vi "Make Config File Body.vi"(0 "VISA resource name":refnum<visa-resource-name>, 11 "error in (no error)":errorcluster) -> (4 "VISA resource name out":refnum<visa-resource-name>, 6 "Result":string, 15 "error out":errorcluster)   [LabVIEW 2020, in "Yokogawa GX Series.lvlib"]
doc: "This VI sets the alarm hysteresis for <B>DX1000/DX2000 series</B>.\nThis VI can be used on Basic Setting Mode at the <B>Set Execution Mode.VI</B>.\n\nAlarm settings on computation channels can be specified on models with the /M1 or /PM1 math option.\nAlarm settings on external input channels can be specified on models with the /MC1 external input channel option."
uses:
  <instrlib>/Yokogawa GX Series/Yokogawa GX Series.lvlib
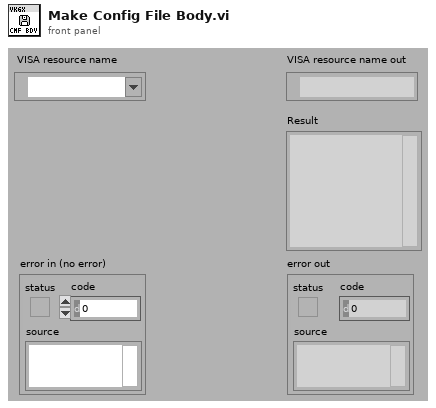
[diagram p1: front panel]
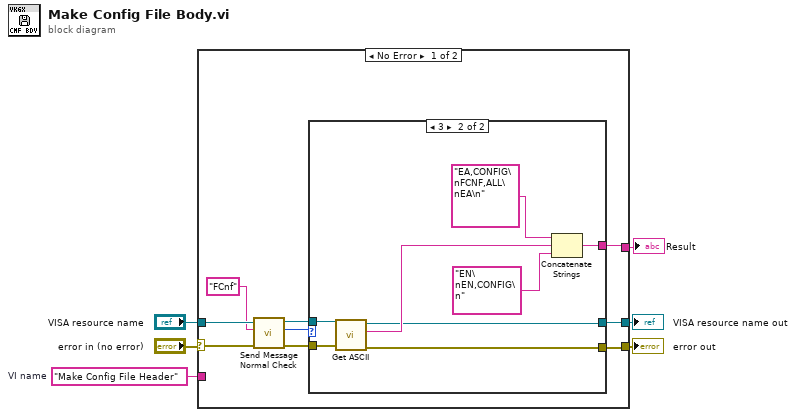
[diagram p0: block diagram]
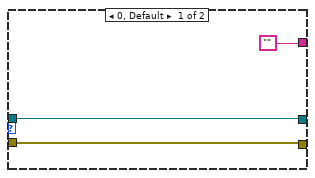
[diagram p2: hidden frame]
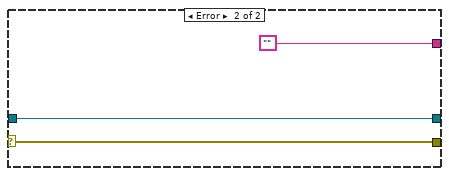
[diagram p3: hidden frame]
diagram:
  w6 = "Make Config File Header"  # VI name
  n1 = case shown="No Error" "error in (no error)" {
    selector: "error in (no error)" -> [w13 w28]
    tunnel: w6 -> [_ _]
    tunnel: [w7 w29] -> w5
    tunnel: [w8 w28] -> w4
    tunnel: [w15 ""] -> w3
    tunnel: "VISA resource name" -> [w14 w29]
    frame No Error {
      n2 = call <instrlib>:"Send Message Normal Check.vi"("error in (no error)"=w13, "Send Message (\"\")"="FCnf", "VISA resource name"=w14) -> ("error out"=w9:errorcluster, "Response Type"=w10:i32, "VISA resource name out"=w11:refnum<visa-resource-name>)  [unwired: 3 in, 3 out]
      n3 = case shown="3" w10 {
        tunnel: ["" w25] -> w15
        tunnel: w11 -> [w18 w24]
        tunnel: w9 -> [w17 w23]
        tunnel: [w17 w20] -> w8
        tunnel: [w18 w19] -> w7
        frame 0, Default {
        }
        frame 3 {
          n4 = call <instrlib>:"Get ASCII.vi"("error in (no error)"=w23, "VISA resource name"=w24) -> ("error out"=w20:errorcluster, "ASCII Data"=w21:string, "VISA resource name out"=w19:refnum<visa-resource-name>)  [unwired: 7 in]
          n5 = Concatenate Strings("EA,CONFIG\nFCNF,ALL\nEA\n", w21, "EN\nEN,CONFIG\n") -> (w25:string)
        }
      }
    }
    frame Error {
    }
  }
  "error out" <- w4
  "VISA resource name out" <- w5
  "Result" <- w3
